vi "Data.Engine.Initialize.vi"(8 "error in":errorcluster, 11 "Custom Device Ref":T1 format="%.0x") -> (0 "error out":errorcluster, 2 "Data Access Engine":refnum<class "Data Access Engine.lvclass">, 3 "Custom Device Ref":T1 format="%.0x")   [LabVIEW 2015, in "Data Access Engine.lvlib" / "Data Access Engine.lvclass"]
uses:
  Data Access Engine.lvclass
  <vilib>/NI Veristand/Custom Device API/Custom Device Item Ref.ctl
  <vilib>/NI Veristand/Custom Device API/Block Data Reference.ctl
  <vilib>/NI Veristand/Custom Device API/Data Reference.ctl
  Data/Read/Read.lvclass
  Data/Write/Write.lvclass
  Data/ReadWrite/ReadWrite.lvclass
  Data Access Engine.lvclass/Data Access Engine.ctl
  <vilib>/NI Veristand/Custom Device API/Get Item Property (Variant).vi
  <vilib>/NI Veristand/Custom Device API/Custom Device API.lvlib
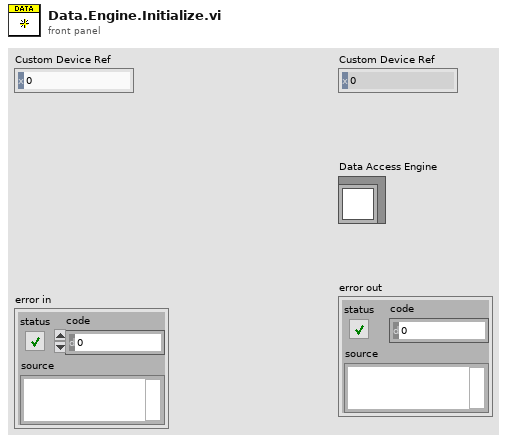
[diagram p1: front panel]
types:
  T1 = typedef "Custom Device API.lvlib/Custom Device Item Ref.ctl" = u64
  T2 = typedef "Custom Device API.lvlib/Block Data Reference.ctl" = cluster{"Data Reference":T3, "Offset":u64, "Length":u64}
  T3 = typedef "Custom Device API.lvlib/Data Reference.ctl" = i32
  T4 = cluster{"Read":cluster{"Refs":T2[], "Values":dbl[]}[], "Write":cluster{"Refs":T3[], "Values":dbl[]}[], "ReadWrite":cluster{"Refs":T3[], "Values":dbl[], "Reset Values":dbl[]}[], "LUT":variant}
  T5 = cluster{"Refs":T3[], "Values":dbl[], "Reset Values":dbl[]}[]
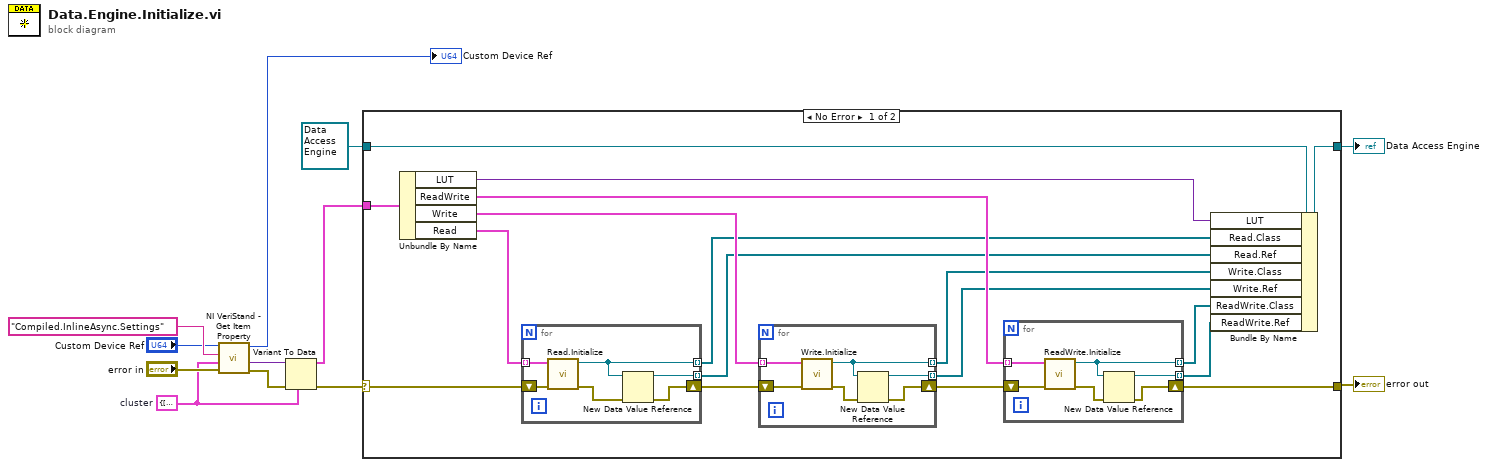
[diagram p0: block diagram]
diagram:
  w8 = T4 {"Read"=[], "Write"=[], "ReadWrite"=[], "LUT"=variant}  # cluster
  n1 = call-poly <vilib>:"NI VeriStand - Get Item Property.vi"("error in (no error)"="error in", "Default Value"=w8, "Property Name"="Compiled.InlineAsync.Settings", "Item Ref in"="Custom Device Ref") -> ("error out"=w11:errorcluster, "Value"=w9:variant, "Item Ref out"=→"Custom Device Ref":T1)  [unwired: 4 in, 1 out]
  n2 = Variant To Data(error in=w11, type=w8, Variant=w9) -> (data=w6:T4, error out=w4:errorcluster)
  n3 = case shown="No Error" w4 {
    selector: w4 -> [w28 w49]
    tunnel: [w25 w49] -> w3
    tunnel: [w19 w48] -> w7
    tunnel: refnum<class "Data Access Engine.lvclass"> refnum ("Data Access API.lvlib:Data Access API.lvclass") -> [w14 w48]
    tunnel: w6 -> [w15 _]
    frame No Error {
      n4 = Unbundle By Name(w15) -> ("LUT"=w13:variant, "ReadWrite"=w23:T5, "Write"=w24:cluster{"Refs":T3[], "Values":dbl[]}[], "Read"=w29:cluster{"Refs":T2[], "Values":dbl[]}[])
      n5 = for {
        tunnel: w29 -> [w47] mode=indexing
        shift-right: [w44] -> w27
        shift-left: w28 -> [w46]
        tunnel: [w43] -> w20 mode=indexing
        tunnel: [w42] -> w16 mode=indexing
        n6 = call "Read.Initialize.vi"("error in (no error)"=w46, "Settings"=w47) -> ("error out"=w45:errorcluster, "Read out"=w43:refnum<class "Read.lvclass">)  [unwired: 8 in]
        n7 = New Data Value Reference(data value=w43, error in=w45) -> (data value reference=w42:refnum<data-value>, error out=w44:errorcluster)
      }
      n8 = for {
        tunnel: w24 -> [w41] mode=indexing
        shift-right: [w37] -> w26
        shift-left: w27 -> [w40]
        tunnel: [w39] -> w21 mode=indexing
        tunnel: [w36] -> w17 mode=indexing
        n9 = call "Write.Initialize.vi"("error in (no error)"=w40, "Settings"=w41) -> ("error out"=w38:errorcluster, "Write out"=w39:refnum<class "Write.lvclass">)  [unwired: 8 in]
        n10 = New Data Value Reference(data value=w39, error in=w38) -> (data value reference=w36:refnum<data-value>, error out=w37:errorcluster)
      }
      n11 = for {
        tunnel: w23 -> [w34] mode=indexing
        shift-right: [w32] -> w25
        shift-left: w26 -> [w35]
        tunnel: [w31] -> w22 mode=indexing
        tunnel: [w30] -> w18 mode=indexing
        n12 = call "ReadWrite.Initialize.vi"("error in (no error)"=w35, "Settings"=w34) -> ("error out"=w33:errorcluster, "ReadWrite out"=w31:refnum<class "ReadWrite.lvclass">)  [unwired: 8 in]
        n13 = New Data Value Reference(data value=w31, error in=w33) -> (data value reference=w30:refnum<data-value>, error out=w32:errorcluster)
      }
      n14 = Bundle By Name(cluster=w14, "LUT"=w13, "Read.Class"=w20, "Read.Ref"=w16, "Write.Class"=w21, "Write.Ref"=w17, "ReadWrite.Class"=w22, "ReadWrite.Ref"=w18) -> (w19:refnum<class "Data Access Engine.lvclass">)
    }
    frame Error {
    }
  }
  "error out" <- w3
  "Data Access Engine" <- w7
